vi "report_gen.vi"(0 "Cantidad de datos":i32, 1 "Grupo":string, 5 "Canal 1":string, 7 "Canal 2":string, 9 "Canal 3":string, 11 "error in (no error)":errorcluster, 12 "Sensor 1":dbl[](array[numeric]), 13 "Sensor 2":dbl[](array[numeric]), 14 "Sensor 3":dbl[](array[numeric])) -> (15 "error out":errorcluster)   [LabVIEW 2025]
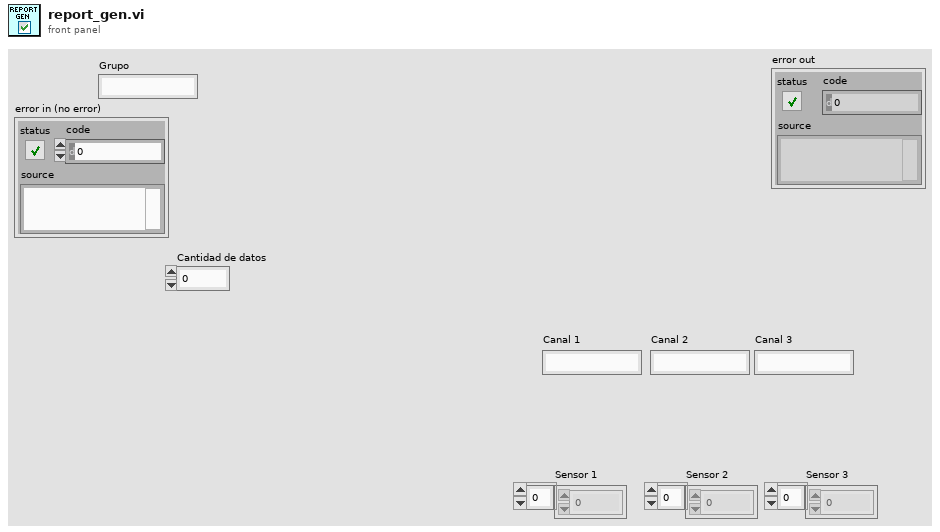
[diagram p1: front panel]
types:
  T1 = enum16{"open", "open or create", "create or replace", "create", "open (read-only)"}
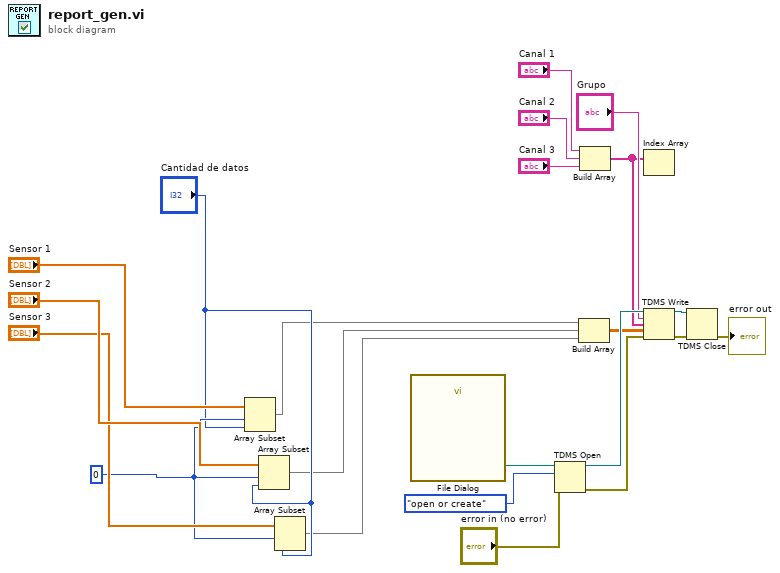
[diagram p0: block diagram]
diagram:
  w6 = 0 ("index")
  n1 = Array Subset(array="Sensor 1", index=w6, length="Cantidad de datos") -> (w4:dbl[])
  n2 = Array Subset(array="Sensor 2", index=w6, length="Cantidad de datos") -> (w3:dbl[])
  n3 = Array Subset(array="Sensor 3", index=w6, length="Cantidad de datos") -> (w2:dbl[])
  n4 = call "File Dialog"() -> ("selected path"=w22:path)  [unwired: 12 in, 3 out]
  n5 = TDMS Open(8:"error in (no error)", 10:T1."open or create" ("operation (0:open)"), 11:w22) -> (0:w18:errorcluster, 3:w20:refnum<k34>)  [unwired: 4 in]
  n6 = Build Array(w4, w3, w2) -> (w1:dbl[][])
  n7 = Build Array("Canal 1", "Canal 2", "Canal 3") -> (w11:string[])
  n8 = Index Array(array=w11) -> ()  [unwired: 1 in, 1 out]
  n9 = TDMS Write(0:w20, 5:"Grupo", 7:w11, 9:w1, 11:w18) -> (4:w15:refnum<k34>, 15:w17:errorcluster)  [unwired: 1 in, 2 out]
  n10 = TDMS Close(8:w17, 11:w15) -> (0:→"error out":errorcluster)  [unwired: 1 out]
